vi "RetrieveWebpage.vi"(4 "lastStringRequired":string, 6 "minimumBytesToRead":i32=3000, 9 "port":u16, 10 "server":string, 11 "pageURL":string) -> (2 "webpageOut":string, 3 "TCPerror":bool)   [LabVIEW 2011]
panel:
  out "actualBytesRequired":i32
  out "loopsRequired":i32
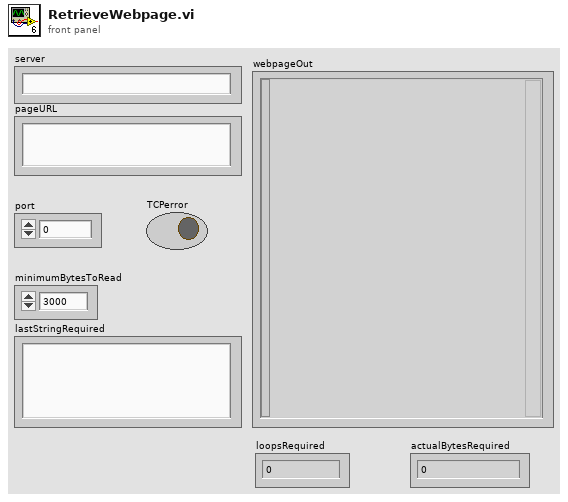
[diagram p1: front panel]
types:
  T1 = enum16{"Standard", "Buffered", "CRLF", "Immediate"}
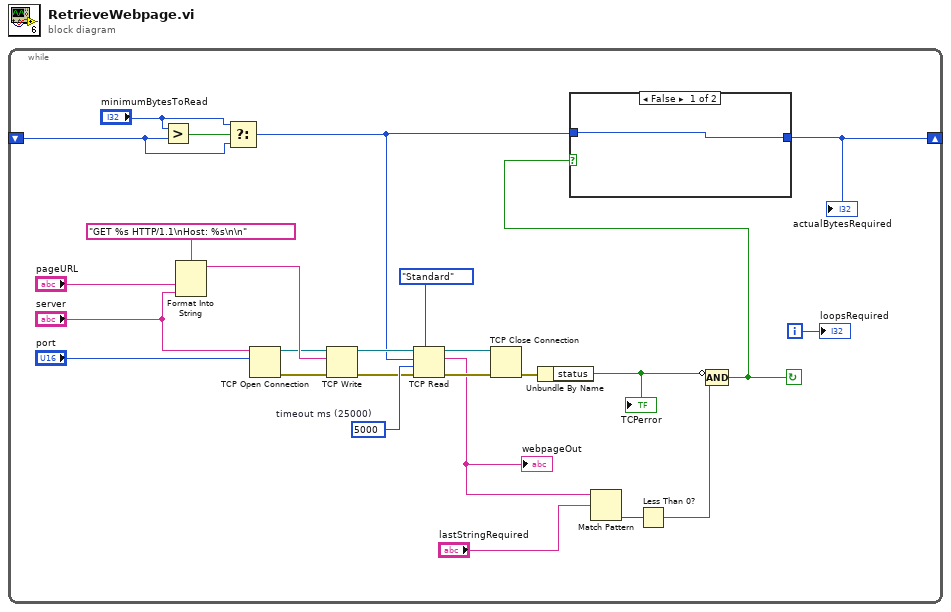
[diagram p0: block diagram]
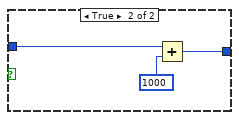
[diagram p2: hidden frame]
diagram:
  n1 = while {
    shift-right: [w8] -> _
    shift-left: _ -> [w9]
    i -> [w1]
    stop <- w2 continue-if-true
    w22 = 5000  # timeout ms (25000)
    n2 = Greater?(x="minimumBytesToRead", y=w9) -> (0:w13:bool)
    n3 = Format Into String(format string="GET %s HTTP/1.1\nHost: %s\n\n" ("data in"), "pageURL", "server") -> (resulting string=w25:string)  [unwired: 2 in, 1 out]
    n4 = Select(t="minimumBytesToRead", s=w13, f=w9) -> (s? t:f=w11:i32)
    n5 = TCP Open Connection(address="server", remote port or service name="port") -> (connection ID=w15:refnum<k5>, error out=w16:errorcluster)  [unwired: 1 in, 2 out]
    n6 = TCP Write(connection ID=w15, data in=w25, error in (no error)=w16) -> (connection ID out=w20:refnum<k5>, error out=w17:errorcluster)  [unwired: 2 out]
    n7 = TCP Read(connection ID=w20, bytes to read=w11, error in (no error)=w17, 7:T1."Standard" ("mode (standard)"), 9:w22) -> (connection ID out=w18:refnum<k5>, data out=w7:string, error out=w19:errorcluster)
    "webpageOut" <- w7
    n8 = TCP Close Connection(connection ID=w18, error in (no error)=w19) -> (error out=w21:errorcluster)  [unwired: 2 out]
    n9 = Unbundle By Name(w21) -> ("status"=w4:bool)
    "TCPerror" <- w4
    n10 = Match Pattern(string=w7, regular expression="lastStringRequired") -> (offset past match=w5:i32)  [unwired: 1 in, 3 out]
    n11 = Less Than 0?(x=w5) -> (x < 0?=w3:bool)
    n12 = Compound Arithmetic op=AND(invert w4, w3) -> (w2:bool)
    n13 = case shown="False" w2 {
      tunnel: w11 -> [w27 w29]
      tunnel: [w27 w28] -> w8
      frame False {
      }
      frame True {
        n14 = Add(x=w29, y=1000 ("x")) -> (x+y=w28:i32)
      }
    }
    "actualBytesRequired" <- w8
    "loopsRequired" <- w1
  }
